vi "Motor Control Enhanced.vi"(0 "PID On":bool=TRUE) -> (5 "Total (V)":dbl[](array[slide])=[5.105602473181425, 4.727577932692882] scale=-8.0..8.0, 6 "Force (N)":T2(graph))   [LabVIEW 2021]
uses:
  <vilib>/Platform/TimedLoop/XDataNode/timing_clust.ctl
  <vilib>/Platform/TimedLoop/XDataNode/nitl_modes.ctl
  <vilib>/Platform/TimedLoop/XDataNode/wakeup.ctl
  <vilib>/DAQmx/write.llb/DAQmx Write (Digital 1D Bool 1Chan 1Samp).vi
  <vilib>/DAQmx/write.llb/DAQmx Write (Analog 1D DBL NChan 1Samp).vi
  <vilib>/DAQmx/create/channels.llb/DAQmx Create Channel (DO-Digital Output).vi
  <vilib>/DAQmx/create/channels.llb/DAQmx Create Channel (AO-Voltage-Basic).vi
  <vilib>/DAQmx/create/channels.llb/DAQmx Create Channel (AI-Voltage-Basic).vi
  <vilib>/DAQmx/miscellaneous.llb/DAQmx Fill In Error Info.vi
  <vilib>/Platform/TimedLoop/XDataNode/XDataNode.xnode
  <vilib>/Platform/TimedLoop/XDataNode/XDNodeRunTimeDep.lvlib
panel:
  in  "Numeric":dbl
  in  "Tab Control":enum32{"PID Gain", "PIN On"}(tab)
  in  "Gains":T1(array[cluster])=[{"proportional gain (Kc)"=0.1, "integral time (Ti, min)"=0.0, "derivative time (Td, min)"=0.0}, {"proportional gain (Kc)"=0.1, "integral time (Ti, min)"=0.0, "derivative time (Td, min)"=0.0}] {"derivative time (Td, min)" format="%.3f"; "integral time (Ti, min)" format="%.3f"; "proportional gain (Kc)" format="%.3f"}
  out "PID (V)":dbl[](array[slide])=[5.105602473181425, 4.727577932692882] scale=-8.0..8.0
  out "Trigger":bool
  out "Position (mm)":cluster{"Position":dbl, "ref_x (mm)":dbl}(graph)
  in  "Loadcell":bool
  in  "Encoder":bool
  out "In Range?":bool
  out "Speed (RPM)":dbl[](array[knob])=[47.6837158203125, 0.0] scale=-200.0..200.0
  out "time (s)":dbl
  in  "Set Point":dbl(slide) scale=0.0..40.0
  in  "Low Limit":bool
  in  "Slope":dbl(slide)=20.0 scale=10.0..30.0
  in  "Floor":dbl(slide)=-3.0
  in  "Motor Enable":bool[](array[boolean])=[FALSE, FALSE]
  in  "stop":bool
  # "FORCE"
  # "TRAJECTORY"
  # "INITIALIZE"
  # "TUNE"
  # "MONITOR"
  # "DEVEL"
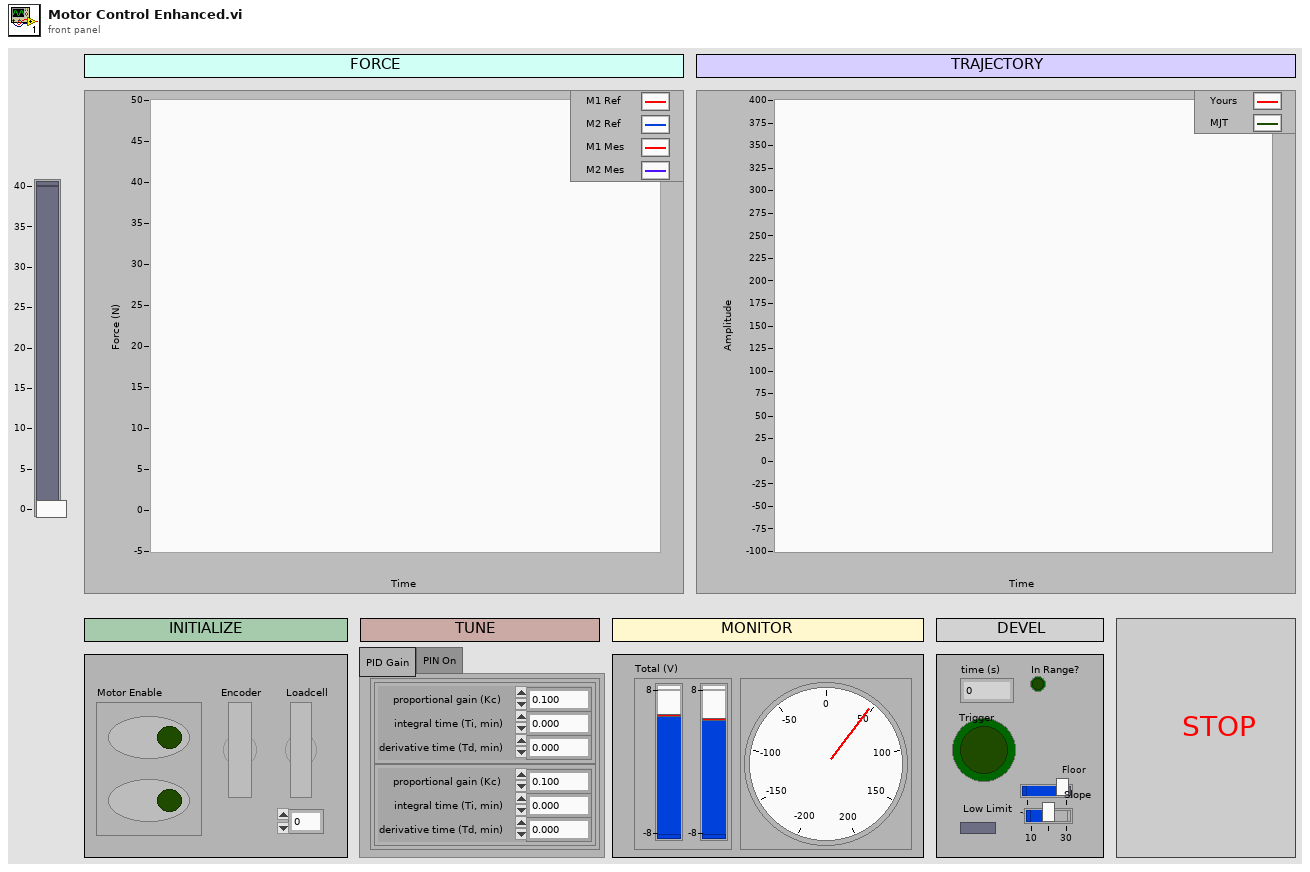
[diagram p1: front panel]
types:
  T1 = cluster{"proportional gain (Kc)":dbl, "integral time (Ti, min)":dbl, "derivative time (Td, min)":dbl}[]
  T2 = cluster{"M1 ref force":dbl, "M2 ref force":dbl, "M1 mes force":dbl, "M2 mes force":dbl}
  T3 = typedef "XDNodeRunTimeDep.lvlib/timing_clust.ctl" = cluster{"Expected End [f-1]":u64, "Actual End [f-1]":u64, "Finished Late? [f-1]":bool, "Expected End [i-1]":u64, "Actual End [i-1]":u64, "Finished Late? [i-1]":bool, "Expected Start [i]":u64, "Actual Start [i]":u64, "Expected Start [f]":u64, "Actual Start [f]":u64, "Source Name":string, "Structure Name":string, "Period":i64, "Deadline":i64, "Offset":i64, "Start":i64, "Priority":i32, "Timeout":i32, "Mode":T4, "Wakeup Reason":T5, "Error":errorcluster, "Source Type":string, "Secondary Source Type":string, "Global End Time":u64, "Global Start Time":u64, "Frame Duration":u64, "Iteration Duration":u64, "Assigned CPU":i32, "I/O Scan Engine Mode":u32}
  T4 = typedef "XDNodeRunTimeDep.lvlib/nitl_modes.ctl" = enum32{"No Change", "Process missed periods, maintain original phase", "Discard missed periods, maintain original phase", "Process missed periods, ignore original phase", "Discard missed periods, ignore original phase"}
  T5 = typedef "XDNodeRunTimeDep.lvlib/wakeup.ctl" = enum32{"Normal", "Aborted", "Asynchronous wakeup", "Timing source error", "Timed loop error", "Timeout"}
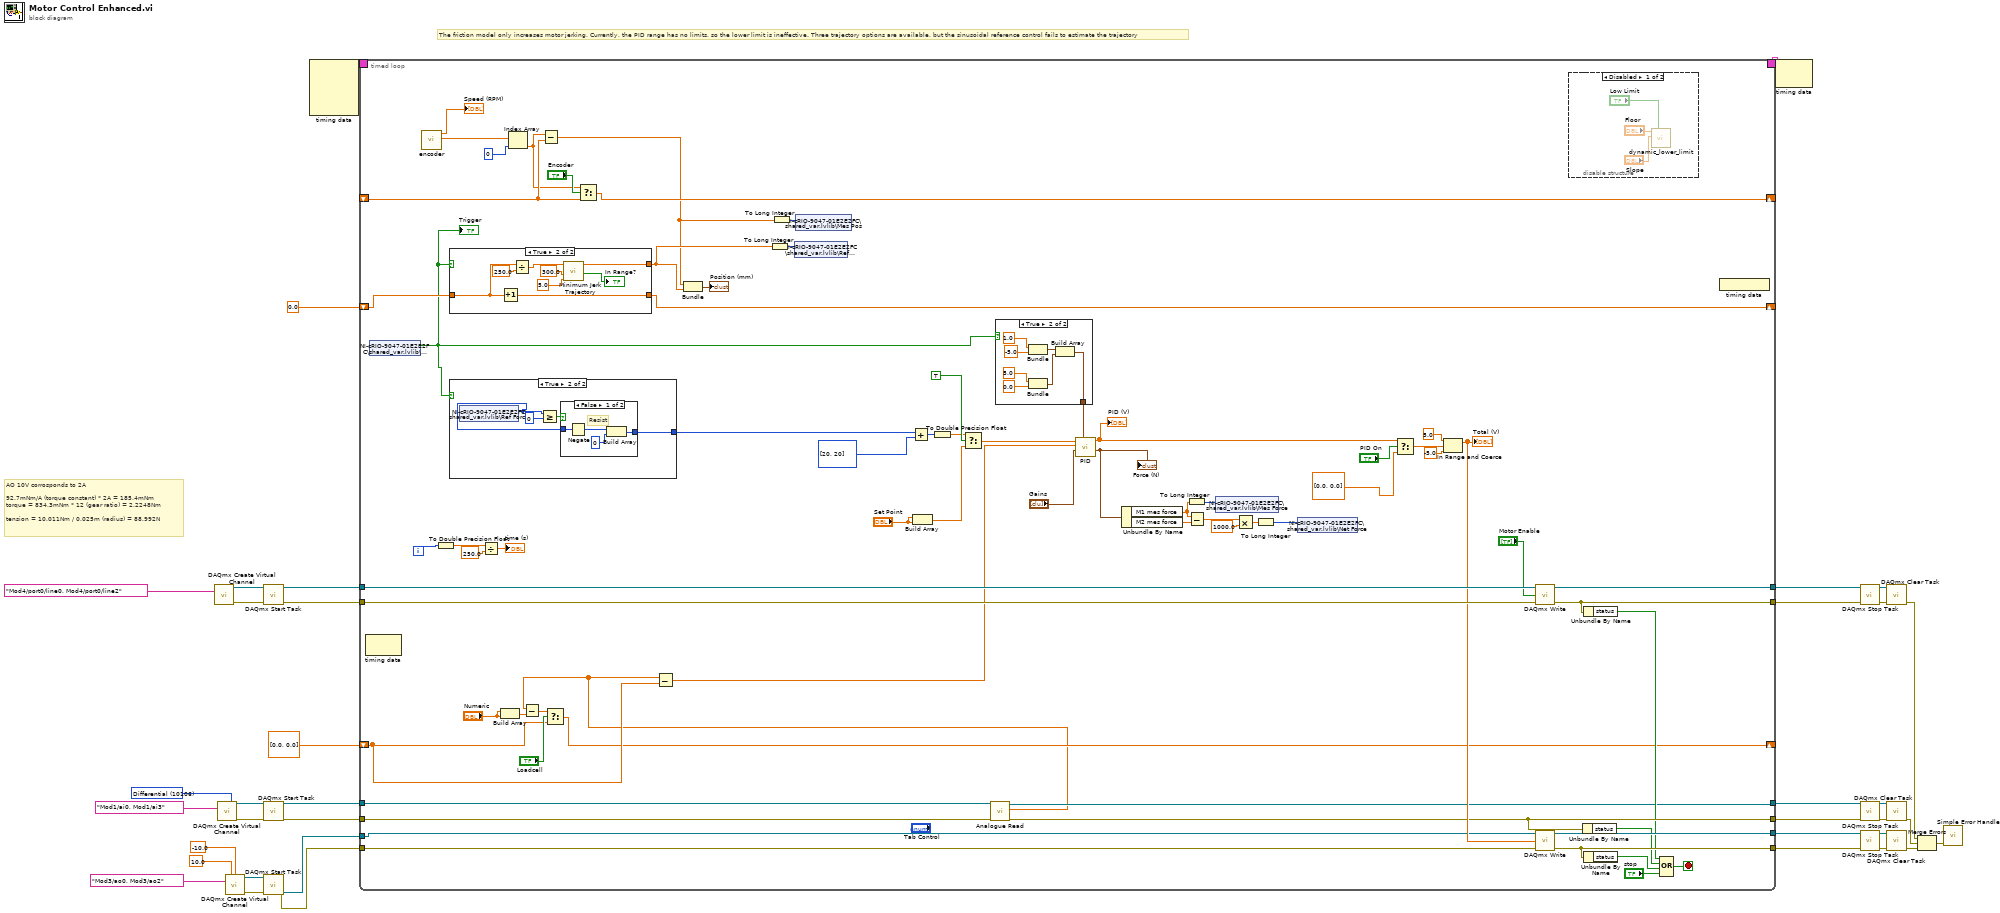
[diagram p0: block diagram]
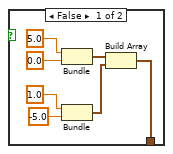
[diagram p3: hidden frame]
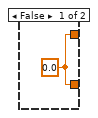
[diagram p4: hidden frame]
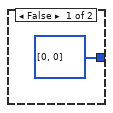
[diagram p5: hidden frame]
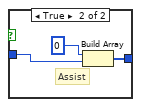
[diagram p6: hidden frame]
diagram:
  w3 = 10106 items=["Default"=-1, "RSE"=10083, "NRSE"=10078, "Differential"=10106, "Pseudodifferential"=12529] ("input terminal configuration")
  # "The friction model only increases motor jerking. Currently, the PID range has no limits, so the lower limit is ineffective. Three trajectory options are available, but the sinusoidal reference control fails to estimate the trajectory"
  # "AO 10V corrosponds to 2A\n\n92.7mNm/A (torque constant) * 2A = 185.4mNm\ntorque = 834.3mNm * 12 (gear ratio) = 2.2248Nm\n\ntension = 10.011Nm / 0.025m (radius) = 88.992N"
  n1 = call-poly <vilib>:"DAQmx Create Virtual Channel.vi"("lines"=tag "Mod4/port0/line0, Mod4/port0/line2") -> ("task out"=w30:refnum<k21>, "error out"=w29:errorcluster)  [unwired: 13 in]
  n2 = call-poly <vilib>:"DAQmx Create Virtual Channel.vi"("input terminal configuration"=w3, "physical channels"=tag "Mod1/ai0, Mod1/ai3") -> ("task out"=w20:refnum<k21>, "error out"=w21:errorcluster)  [unwired: 12 in]
  n3 = call-poly <vilib>:"DAQmx Create Virtual Channel.vi"("maximum value"=10.0 ("AO max"), "minimum value"=-10.0 ("AO min"), "physical channels"=tag "Mod3/ao0, Mod3/ao2" ("Physical Channel(s)")) -> ("task out"=w14:refnum<k21>, "error out"=w13:errorcluster)  [unwired: 11 in]
  n4 = call <vilib>:"DAQmx Start Task.vi"("task/channels in"=w30, "error in"=w29) -> ("task out"=w27:refnum<k21>, "error out"=w26:errorcluster)  [unwired: 12 in]
  n5 = call <vilib>:"DAQmx Start Task.vi"("task/channels in"=w20, "error in"=w21) -> ("task out"=w18:refnum<k21>, "error out"=w17:errorcluster)  [unwired: 12 in]
  n6 = call <vilib>:"DAQmx Start Task.vi"("task/channels in"=w14, "error in"=w13) -> ("task out"=w32:refnum<k21>, "error out"=w31:errorcluster)  [unwired: 12 in]
  n7 = node-c288() -> (w34:T3)  [unwired: 4 in]
  n8 = timed-loop {
    tunnel: [w108] -> w38
    tunnel: [w107] -> w37
    tunnel: [w65] -> w36
    tunnel: [w94] -> w35
    tunnel: w18 -> [w105]
    timing: w34 -> [_]
    timing-out: [_] -> w33
    tunnel: w17 -> [w104]
    tunnel: w32 -> [w64]
    tunnel: w31 -> [w106]
    tunnel: w27 -> [w103]
    tunnel: w26 -> [w102]
    tunnel: [w101] -> w23
    tunnel: [w95] -> w22
    shift-right: [w76] -> _
    shift-left: 0.0 ("total time") -> [w77]
    shift-right: [w71] -> _
    shift-left: _ -> [w69]
    shift-right: [w50] -> _
    shift-left: dbl[] [0.0, 0.0] ("measured force") -> [w51]
    i -> [w82]
    stop <- w90 stop-if-true
    n9 = node-c288() -> ()  [unwired: 1 in, 1 out]
    n10 = shared-variable "NI-cRIO-9047-01E2E2FC\\shared_var.lvlib\\Trigger"() -> (w43:bool)  [unwired: 1 in, 1 out]
    "Trigger" <- w43
    n11 = call "encoder.vi"() -> ("Mes Pos (mm)"=w74:dbl[], "RPM"=→"Speed (RPM)":dbl[])  [unwired: 10 in]
    n12 = To Double Precision Float(number=w82) -> (double precision float=w81:dbl)
    n13 = case shown="True" w43 {
      tunnel: w77 -> [_ w130]
      tunnel: [w128 w133] -> w76
      tunnel: [w128 w129] -> w61
      frame False {
        w128 = 0.0
      }
      frame True {
        n14 = Increment(x=w130) -> (x+1=w133:dbl)
        n15 = Divide(x=w130, y=250.0) -> (x/y=w131:dbl)
        n16 = call "Minimum Jerk Trajectory.vi"("total time"=5.0, "total length"=300.0, "t (sec)"=w131) -> ("In Range?"=→"In Range?":bool, "ref_x (mm)"=w129:dbl)  [unwired: 7 in]
      }
    }
    n17 = case shown="True" w43 {
      tunnel: [i32[] [0, 0] w141] -> w67
      frame False {
      }
      frame True {
        n18 = shared-variable "NI-cRIO-9047-01E2E2FC\\shared_var.lvlib\\Ref Force"() -> (w140:i32)  [unwired: 1 in, 1 out]
        n19 = Greater Or Equal?(x=w140, y=0) -> (x >= y?=w138:bool)
        n20 = case shown="False" w138 {
          tunnel: w140 -> [w144 w147]
          tunnel: [w145 w148] -> w141
          frame False {
            # "Resist"
            n21 = Negate(x=w144) -> (-x=w142:i32)
            n22 = Build Array(w142, 0 ("element")) -> (w145:i32[])
          }
          frame True {
            # "Assist"
            n23 = Build Array(0 ("element"), w147) -> (w148:i32[])
          }
        }
      }
    }
    n24 = Divide(x=w81, y=250.0) -> (x/y=→"time (s)":dbl)
    n25 = Build Array("Numeric", "Numeric") -> (w39:dbl[])
    n26 = Index Array(array=w74, index=0) -> (element=w68:dbl)
    n27 = Subtract(x=w68, y=w69) -> (x-y=w60:dbl)
    n28 = Select(t=w68, s="Encoder", f=w69) -> (s? t:f=w71:dbl)
    n29 = Bundle(w60, "ref_x (mm)"=w61) -> (→"Position (mm)":cluster{dbl, "ref_x (mm)":dbl})  [unwired: 1 in]
    n30 = To Long Integer(number=w61) -> (32bit integer=w46:i32)
    n31 = To Long Integer(number=w60) -> (32bit integer=w45:i32)
    n32 = shared-variable "NI-cRIO-9047-01E2E2FC\\shared_var.lvlib\\Ref Pos"(w46) -> ()  [unwired: 1 in, 1 out]
    n33 = shared-variable "NI-cRIO-9047-01E2E2FC\\shared_var.lvlib\\Mes Pos"(w45) -> ()  [unwired: 1 in, 1 out]
    n34 = Add(x=w67, y=i32[] [20, 20] ("x")) -> (x+y=w63:i32[])
    n35 = Build Array("Set Point", "Set Point") -> (w84:dbl[])
    n36 = To Double Precision Float(number=w63) -> (double precision float=w62:dbl[])
    n37 = Select(t=w62, s=TRUE, f=w84) -> (s? t:f=w57:dbl[])
    n38 = call "Analogue Read.vi"("error in"=w104, "task/channels in"=w105) -> ("error out"=w94:errorcluster, "measured force"=w48:dbl[], "task out"=w65:refnum<k21>)  [unwired: 6 in, 1 out]
    n39 = Subtract(x=w48, y=w39) -> (x-y=w47:dbl[])
    n40 = Select(t=w47, s="Loadcell", f=w51) -> (s? t:f=w50:dbl[])
    n41 = Subtract(x=w48, y=w51) -> (x-y=w49:dbl[])
    n42 = case shown="True" w43 {
      tunnel: [w114 w121] -> w53
      frame False {
        n43 = Bundle(5.0, 0.0) -> (w120:cluster{dbl, dbl})  [unwired: 1 in]
        n44 = Bundle(1.0, -5.0) -> (w119:cluster{dbl, dbl})  [unwired: 1 in]
        n45 = Build Array(w120, w119) -> (w114:cluster{dbl, dbl}[])
      }
      frame True {
        n46 = Bundle(1.0, -5.0) -> (w122:cluster{dbl, dbl})  [unwired: 1 in]
        n47 = Bundle(5.0, 0.0) -> (w123:cluster{dbl, dbl})  [unwired: 1 in]
        n48 = Build Array(w122, w123) -> (w121:cluster{dbl, dbl}[])
      }
    }
    n49 = call "PID.vi"("output range"=w53, "PID gains"="Gains", "mes force"=w49, "ref force"=w57) -> ("output cluster"=w41:T2, "PID output"=w88:dbl[])  [unwired: 6 in]
    "Force (N)" <- w41
    "PID (V)" <- w88
    n50 = Unbundle By Name(w41) -> ("M1 mes force"=w54:dbl, "M2 mes force"=w55:dbl)
    n51 = To Long Integer(number=w54) -> (32bit integer=w56:i32)
    n52 = Subtract(x=w54, y=w55) -> (x-y=w59:dbl)
    n53 = shared-variable "NI-cRIO-9047-01E2E2FC\\shared_var.lvlib\\Mes Force"(w56) -> ()  [unwired: 1 in, 1 out]
    n54 = Multiply(x=w59, y=1000.0) -> (x*y=w42:dbl)
    n55 = To Long Integer(number=w42) -> (32bit integer=w44:i32)
    n56 = shared-variable "NI-cRIO-9047-01E2E2FC\\shared_var.lvlib\\Net Force"(w44) -> ()  [unwired: 1 in, 1 out]
    n57 = Select(t=w88, s="PID On", f=dbl[] [0.0, 0.0]) -> (s? t:f=w86:dbl[])
    n58 = In Range and Coerce(upper limit=5.0, x=w86, lower limit=-5.0) -> (coerced(x)=w96:dbl[])  [unwired: 1 out]
    "Total (V)" <- w96
    n59 = call-poly <vilib>:"DAQmx Write.vi"("task/channels in"=w103, "data"="Motor Enable", "error in"=w102) -> ("task out"=w101:refnum<k21>, "error out"=w95:errorcluster)  [unwired: 10 in, 1 out]
    n60 = call-poly <vilib>:"DAQmx Write.vi"("task/channels in"=w64, "data"=w96, "error in"=w106) -> ("task out"=w108:refnum<k21>, "error out"=w107:errorcluster)  [unwired: 10 in, 1 out]
    n61 = disable-structure shown="Disabled" {
      frame Disabled {
        n62 = call "dynamic_lower_limit.vi"("Boolean"="Low Limit", "v_max"="Slope", "F_L"="Floor") -> ()  [unwired: 8 in, 1 out]
      }
      frame Enabled {
      }
    }
    n63 = Unbundle By Name(w94) -> ("status"=w92:bool)
    n64 = Unbundle By Name(w95) -> ("status"=w91:bool)
    n65 = Unbundle By Name(w107) -> ("status"=w93:bool)
    n66 = Compound Arithmetic op=OR(w91, w92, w93, "stop") -> (w90:bool)
    n67 = node-c288() -> ()  [unwired: 1 out]
  }
  n68 = node-c288(w33) -> ()  [unwired: 1 out]
  n69 = call <vilib>:"DAQmx Stop Task.vi"("task/channels in"=w23, "error in"=w22) -> ("task out"=w25:refnum<k21>, "error out"=w24:errorcluster)  [unwired: 12 in]
  n70 = call <vilib>:"DAQmx Stop Task.vi"("task/channels in"=w36, "error in"=w35) -> ("task out"=w9:refnum<k21>, "error out"=w8:errorcluster)  [unwired: 12 in]
  n71 = call <vilib>:"DAQmx Stop Task.vi"("task/channels in"=w38, "error in"=w37) -> ("task out"=w11:refnum<k21>, "error out"=w10:errorcluster)  [unwired: 12 in]
  n72 = call <vilib>:"DAQmx Clear Task.vi"("task in"=w25, "error in"=w24) -> ("error out"=w4:errorcluster)  [unwired: 13 in]
  n73 = call <vilib>:"DAQmx Clear Task.vi"("task in"=w9, "error in"=w8) -> ("error out"=w5:errorcluster)  [unwired: 13 in]
  n74 = call <vilib>:"DAQmx Clear Task.vi"("task in"=w11, "error in"=w10) -> ("error out"=w6:errorcluster)  [unwired: 13 in]
  n75 = Merge Errors(w4, w5, w6) -> (w7:errorcluster)
  n76 = call <vilib>:"Simple Error Handler.vi"("error in (no error)"=w7) -> ()  [unwired: 4 in, 5 out]
